vi "observacao_0MQ.vi"() -> ()   [LabVIEW 2012, in "Shared_160.lvlib"] (continued)
                n700 = call "Monta Comando.vi"("Comando"="PARAR", "Dispositivo"="PROG" ("Comando"), "Controlador"=w605) -> ()  [unwired: 4 in, 3 out]
              }
              frame 4 {
                w608 = u16 7 items=["Alarme", "Atencao", "Erro", "Ocupado", "TBD", "LCB", "Trapeira", "Paravento", "DomoRap", "DomoCW", "DomoCCW", "TBD", "Em movimento", "TBD"] ("NomeStatus")
                # "Verifica Paravento"
                n701 = call "Bit Status CUP.vi"("NomeStatus"=w608) -> ("StatBit"=w612:bool)
                n702 = Not(x=w612) -> (.not. x?=w613:bool)
                n703 = And(x=w613, y="ChkWindDown") -> (x .and. y?=w610:bool)
                n704 = case shown="True" w610 {
                  tunnel: w609 -> [_ w616]
                  tunnel: [6 w615] -> w607
                  frame False {
                    # "Paravento abaixado\nou desabilitado"
                  }
                  frame True {
                    # "Descer Parav."
                    n705 = case shown="True" w616 {
                      tunnel: [5 w621] -> w615
                      frame False {
                        w620 = u16 4 items=["ZERO", "AH", "DEC", "TUBO", "CUP"] ("Controlador")
                        # "Aguardar abaixa/o Parav."
                        # "CLP Pronto"
                        n706 = call "Monta Comando.vi"("Comando"="DESCER", "Dispositivo"="PARAVENTO" ("Comando"), "Controlador"=w620) -> ()  [unwired: 4 in, 3 out]
                      }
                      frame True {
                        # "CLP Busy"
                        n707 = local read "TimeoutCUP"() -> (w623:u32)
                        n708 = call "TickTimeout.vi"("msInicial"=w623, "msTimeout"=u32 5000) -> ("Timeout"=w622:bool)  [unwired: 2 out]
                        n709 = case shown="True" w622 {
                          tunnel: [4 3] -> w621
                          frame False {
                          }
                          frame True {
                          }
                        }
                      }
                    }
                  }
                }
              }
              frame 5 {
                w627 = u16 7 items=["Alarme", "Atencao", "Erro", "Ocupado", "TBD", "LCB", "Trapeira", "Paravento", "DomoRap", "DomoCW", "DomoCCW", "TBD", "Em movimento", "TBD"] ("NomeStatus")
                # "Aqui também caberia um Timeout?"
                # "Também poderia ser testado o bit \"Em movimento\".\nNeste caso o código do \"IF\" deve ser permutado."
                # "Aguarda abaixamento Paravento"
                n710 = call "Bit Status CUP.vi"("NomeStatus"=w627) -> ("StatBit"=w629:bool)
                n711 = case shown="True" w629 {
                  tunnel: [5 6] -> w628
                  frame False {
                    # "Ainda movendo...\nAGUARDAR"
                  }
                  frame True {
                    # "Paravento abaixado."
                  }
                }
              }
              frame 6 {
                w632 = u16 6 items=["Alarme", "Atencao", "Erro", "Ocupado", "TBD", "LCB", "Trapeira", "Paravento", "DomoRap", "DomoCW", "DomoCCW", "TBD", "Em movimento", "TBD"] ("NomeStatus")
                # "Verifica Trapeira"
                n712 = call "Bit Status CUP.vi"("NomeStatus"=w632) -> ("StatBit"=w633:bool)
                n713 = Not(x=w633) -> (.not. x?=w637:bool)
                n714 = And(x=w637, y="ChkOpenShutter") -> (x .and. y?=w635:bool)
                n715 = case shown="False" w635 {
                  tunnel: [0 w642] -> w638
                  tunnel: w634 -> [_ w643]
                  frame False {
                    # "Verificar Paravento"
                    # "Trapeira aberta\nou desabilitada"
                    n716 = call "TickTimeout.vi"() -> ("msTick"=w639:u32)  [unwired: 2 in, 2 out]
                    n717 = local write "TimeoutCUP"(w639) -> ()
                    n718 = global write "Global_Telescopio.vi" "T cup"(w639) -> ()
                    "Dome on Target" <- TRUE
                  }
                  frame True {
                    # "Abrir Trapeira"
                    n719 = case shown="False" w643 {
                      tunnel: [7 w648] -> w642
                      frame False {
                        w647 = u16 4 items=["ZERO", "AH", "DEC", "TUBO", "CUP"] ("Controlador")
                        # "Aguardar abertura Trap."
                        # "CLP Pronto"
                        n720 = call "Monta Comando.vi"("Comando"="ABRIR", "Dispositivo"="TRAPEIRA" ("Comando"), "Controlador"=w647) -> ()  [unwired: 4 in, 3 out]
                      }
                      frame True {
                        # "CLP Busy"
                        n721 = local read "TimeoutCUP"() -> (w650:u32)
                        n722 = call "TickTimeout.vi"("msInicial"=w650, "msTimeout"=u32 5000) -> ("Timeout"=w649:bool)  [unwired: 2 out]
                        n723 = case shown="True" w649 {
                          tunnel: [6 3] -> w648
                          frame False {
                          }
                          frame True {
                          }
                        }
                      }
                    }
                  }
                }
              }
              frame 7 {
                w654 = u16 6 items=["Alarme", "Atencao", "Erro", "Ocupado", "TBD", "LCB", "Trapeira", "Paravento", "DomoRap", "DomoCW", "DomoCCW", "TBD", "Em movimento", "TBD"] ("NomeStatus")
                # "Aqui também caberia um Timeout?"
                # "Aguarda abertura Trapeira"
                # "Também poderia ser testado o bit \"Em movimento\".\nNeste caso o código do \"IF\" deve ser permutado."
                n724 = call "Bit Status CUP.vi"("NomeStatus"=w654) -> ("StatBit"=w655:bool)
                n725 = case shown="True" w655 {
                  tunnel: [7 0] -> w656
                  frame False {
                    # "Ainda movendo...\nAGUARDAR"
                  }
                  frame True {
                    w659 = TRUE ("Dome on Target")
                    # "Trapeira aberta.\nFIM"
                    n726 = call "TickTimeout.vi"() -> ("msTick"=w658:u32)  [unwired: 2 in, 2 out]
                    n727 = local write "Dome on Target"(w659) -> ()
                    n728 = local write "RefreshShutterState"(w659) -> ()
                    n729 = local write "TimeoutCUP"(w658) -> ()
                    n730 = global write "Global_Telescopio.vi" "T cup"(w658) -> ()
                  }
                }
              }
            }
            n731 = And(x=w523, y=w508) -> (x .and. y?=w519:bool)
            n732 = case shown="True" w519 {
              tunnel: w508 -> [w537 _]
              tunnel: [w536 "POINT" ("Boolean Text.Text")] -> w507
              frame False {
                n733 = case shown="True" w537 {
                  tunnel: ["POINT" ("Boolean Text.Text") "STOP" ("Boolean Text.Text")] -> w536
                  frame False {
                  }
                  frame True {
                  }
                }
              }
              frame True {
                w540 = TRUE
                # "MUDANÇA:\n22/6/2011 \nHab. Guider"
                n734 = local read "ChkDomeEnable"() -> (w541:bool)
                n735 = global write "Global_Telescopio.vi" "Botão GO = STOP"(FALSE) -> ()
                n736 = local write "LED GUIDER"(w540) -> ()
                n737 = local write "GUIDER"(w540) -> ()
                n738 = local write "DOME"(w541) -> ()
              }
            }
            n739 = Tick Count (ms)() -> (millisecond timer value=w500:u32)
            n740 = Subtract(x=w500, y=w506) -> (x-y=w499:u32)
            n741 = Less?(x=w499, y=w501) -> (x < y?=w502:bool)
            n742 = case shown="True" w502 {
              tunnel: w501 -> [_ w535]
              frame False {
              }
              frame True {
                n743 = Wait Until Next ms Multiple(millisecond multiple=w535) -> ()  [unwired: 1 out]
              }
            }
            n744 = control-ref of="BtTargetPoint"() -> (w534:refnum<vi>)
            n745 = call "PROTECAO.vi"("Estado In"=w512) -> ("Estado Out"=w511:i32)  [unwired: 2 in]
            n746 = property class="Bool"(reference=w534, "Boolean Text.Text"=w507) -> ()  [unwired: 1 in, 2 out]
            n747 = local write "statCUP"(w511) -> ()
            "statCUP 2" <- "statCUP"
            "Erro Lim" <- 15 ("y")
            "Erro PROTEC" <- 10 ("y")
          }
          frame #4 {
            # "CHECA FINAL DO APONTAMENTO"
            # "ascensão reta = tempo sideral - ângulo horário (2)"
            n748 = local read "LedPointing"() -> (w957:bool)
            n749 = case shown="True" w957 {
              frame False {
                n750 = property on="DOME" class="Bool (strict)"("Disabled"=u8 0) -> ()  [unwired: 2 in, 2 out]
              }
              frame True {
                n751 = local read "statCUP"() -> (w962:i32)
                n752 = local read "statAH"() -> (w961:i32)
                n753 = local read "statDEC"() -> (w963:i32)
                n754 = Compound Arithmetic op=ADD(w962, w961, w963) -> (w964:i32)
                n755 = Greater Than 0?(x=w964) -> (x > 0?=w960:bool)
                n756 = case shown="False" w960 {
                  selector: w960 -> [w965 _]
                  frame False {
                    w968 = TRUE
                    n757 = local read "ChkPointPrecessed"() -> (w966:bool)
                    n758 = local read "StrPointObjName"() -> (w971:string)
                    n759 = local read "StrPointObjRA"() -> (w970:string)
                    n760 = local read "StrPointObjDEC"() -> (w969:string)
                    n761 = local write "LedPointing"(w965) -> ()
                    n762 = property on="LedPointing" class="Bool (strict)"("Visible"=w965) -> ()  [unwired: 2 in, 2 out]
                    n763 = case shown="True" w966 {
                      tunnel: ["2000.000000000" ("Saída") w973] -> w967
                      frame False {
                        # "20240805"
                      }
                      frame True {
                        # "20240805"
                        n764 = call "Calcula epoch.vi"() -> ("epoch"=w976:dbl)  [unwired: 2 in]
                        n765 = Number To Fractional String(number=w976, precision (6)=i16 9) -> (F-format string=w974:string)  [unwired: 2 in]
                        n766 = call "Comma_to_Point.vi"("Lat_A"=w974) -> ("Saída"=w973:string)
                      }
                    }
                    n767 = global write "Global_Telescopio.vi" "NAME OBJETO"(w971) -> ()
                    n768 = global write "Global_Telescopio.vi" "DEC AQUIS"(w969) -> ()
                    n769 = global write "Global_Telescopio.vi" "RA AQUIS"(w970) -> ()
                    n770 = local write "Processa Centragem"(w968) -> ()
                    n771 = property on="LedPointWorkArea" class="Bool (strict)"("Visible"=w968) -> ()  [unwired: 2 in, 2 out]
                    n772 = global write "Global_Telescopio.vi" "EPOCH AQUIS"(w967) -> ()
                  }
                  frame True {
                  }
                }
              }
            }
            n773 = local read "VARIABLE \nTRACKING"() -> (w958:bool)
            n774 = case shown="True" w958 {
              frame False {
              }
              frame True {
                n775 = local write "DEC"("DECTARGET") -> ()
                n776 = local write "RA"("AHTARGET") -> ()
              }
            }
          }
          frame #5 {
            # "PROCESSO OBJETO CENTRADO"
            n777 = case shown="True" "Processa Centragem" {
              frame False {
              }
              frame True {
                w985 = u16 3 items=["Alarme", "Atencao", "Erro", "Ocupado", "Protecao", "Embreagem", "Tracking", "Var. Track", "Rápido", "Ligeiro", "Médio", "Lento", "Em movimento", ""] ("NomeStatus")
                w986 = u16 3 items=["Alarme", "Atencao", "Erro", "Ocupado", "Protecao", "Embreagem", "Tracking", "Var. Track", "Rápido", "Ligeiro", "Médio", "Lento", "Em movimento", ""] ("NomeStatus")
                # "Roda case interno quando \nos controladores AH e DEC\nestiverem desocupados."
                n778 = call "Bit Status AH.vi"("NomeStatus"=w986) -> ("StatBit"=w984:bool)
                n779 = call "Bit Status DEC.vi"("NomeStatus"=w985) -> ("StatBit"=w983:bool)
                n780 = Or(x=w984, y=w983) -> (x .or. y?=w980:bool)
                n781 = case shown="False" w980 {
                  selector: w980 -> [w1005 _]
                  tunnel: "INDEXER" ("Comando") -> [w1007 _]
                  tunnel: "ZERAR" ("Comando") -> [w1006 _]
                  frame False {
                    w993 = u16 1 items=["ZERO", "AH", "DEC", "TUBO", "CUP"] ("Controlador")
                    w994 = u16 2 items=["ZERO", "AH", "DEC", "TUBO", "CUP"] ("Controlador")
                    w987 = 0.0 ("AcumAG DEC")
                    # "PROCESSOPRECESSÃO"
                    # "PROCESSO ZERA POS_MOTOR"
                    # "Precessão"
                    n782 = local read "PM_RA"() -> (w999:string)
                    n783 = local read "Temp amb"() -> (w1002:string)
                    n784 = local read "hum local"() -> (w1000:string)
                    n785 = local read "MeanDEC"() -> (w1003:string)
                    n786 = local read "pressão atm"() -> (w1001:string)
                    n787 = local read "MeanRA"() -> (w1004:string)
                    n788 = local read "PM_DEC"() -> (w998:string)
                    n789 = call "Monta Comando.vi"("Comando"=w1006, "Dispositivo"=w1007, "Controlador"=w993) -> ()  [unwired: 4 in, 3 out]
                    n790 = call "Monta Comando.vi"("Comando"=w1006, "Dispositivo"=w1007, "Controlador"=w994) -> ()  [unwired: 4 in, 3 out]
                    n791 = call "PrecessFortran.vi"("Asc reta"=w1004, "Var RA"=w999, "Declinação"=w1003, "Temperatura (Kelvin)"=w1002, "Pressao atmosferica (mB)"=w1001, "Humidade relativa (0 a 1)"=w1000, "Var DEC"=w998) -> ("Observed RA (radians)"=w997:dbl, "Observed Dec (radians)"=w996:dbl)  [unwired: 2 in, 5 out]
                    n792 = local write "Processa Centragem"(w1005) -> ()
                    n793 = global write "Global_Telescopio.vi" "LatchPrecRA"(w997) -> ()
                    n794 = global write "Global_Telescopio.vi" "LatchPrecDEC"(w996) -> ()
                    n795 = global read "Global_Telescopio.vi" "Sideral Time"() -> (w990:dbl)
                    n796 = global read "Global_Telescopio.vi" "PosDEC"() -> (w992:dbl)
                    n797 = global read "Global_Telescopio.vi" "PosAH"() -> (w991:dbl)
                    n798 = Subtract(x=w990, y=w991) -> (x-y=w989:dbl)
                    n799 = local write "LatchDeslocDEC"(w992) -> ()
                    n800 = local write "LatchDeslocRA"(w989) -> ()
                    n801 = global write "Global_Telescopio.vi" "AcumPrecDEC"(w987) -> ()
                    n802 = global write "Global_Telescopio.vi" "LatchAG RA"(w987) -> ()
                    n803 = global write "Global_Telescopio.vi" "AcumAG DEC"(w987) -> ()
                    n804 = global write "Global_Telescopio.vi" "AcumPrecRA"(w987) -> ()
                    n805 = global write "Global_Telescopio.vi" "LatchAG DEC"(w987) -> ()
                    n806 = global write "Global_Telescopio.vi" "AcumAG RA"(w987) -> ()
                    n807 = global write "Global_Telescopio.vi" "ObjCentrado"(TRUE) -> ()
                    n808 = property on="Calagem" class="Bool"("Disabled"=u8 0) -> ()  [unwired: 2 in, 2 out]
                  }
                  frame True {
                  }
                }
              }
            }
          }
          frame #6 {
            w1011 = u16 2 items=["Alarme", "Atencao", "Erro", "Ocupado", "TBD", "LCB", "Trapeira", "Paravento", "DomoRap", "DomoCW", "DomoCCW", "TBD", "Em movimento", "TBD"] ("NomeStatus")
            w1012 = u16 3 items=["Alarme", "Atencao", "Erro", "Ocupado", "TBD", "LCB", "Trapeira", "Paravento", "DomoRap", "DomoCW", "DomoCCW", "TBD", "Em movimento", "TBD"] ("NomeStatus")
            w1016 = u16 3 items=["Alarme", "Atencao", "Erro", "Ocupado", "Protecao", "Embreagem", "Tracking", "Var. Track", "Rápido", "Ligeiro", "Médio", "Lento", "Em movimento", ""] ("NomeStatus")
            w1017 = u16 3 items=["Alarme", "Atencao", "Erro", "Ocupado", "Protecao", "Embreagem", "Tracking", "Var. Track", "Rápido", "Ligeiro", "Médio", "Lento", "Em movimento", ""] ("NomeStatus")
            w1025 = "ERROS" ("Comando")
            w1028 = u16 2 items=["Alarme", "Atencao", "Erro", "Ocupado", "Protecao", "Embreagem", "Tracking", "Var. Track", "Rápido", "Ligeiro", "Médio", "Lento", "Em movimento", ""] ("NomeStatus")
            w1029 = u16 2 items=["Alarme", "Atencao", "Erro", "Ocupado", "Protecao", "Embreagem", "Tracking", "Var. Track", "Rápido", "Ligeiro", "Médio", "Lento", "Em movimento", ""] ("NomeStatus")
            w1026 = "PROG" ("Comando")
            # "LOGTCS ERROS"
            n809 = call "Bit Status AH.vi"("NomeStatus"=w1029) -> ("StatBit"=w1019:bool)
            n810 = call "Bit Status AH.vi"("NomeStatus"=w1017) -> ("StatBit"=w1015:bool)
            n811 = call "Bit Status DEC.vi"("NomeStatus"=w1028) -> ("StatBit"=w1018:bool)
            n812 = call "Bit Status DEC.vi"("NomeStatus"=w1016) -> ("StatBit"=w1014:bool)
            n813 = call "Bit Status CUP.vi"("NomeStatus"=w1011) -> ("StatBit"=w1027:bool)
            n814 = call "Bit Status CUP.vi"("NomeStatus"=w1012) -> ("StatBit"=w1024:bool)
            n815 = Not(x=w1024) -> (.not. x?=w1023:bool)
            n816 = Not(x=w1015) -> (.not. x?=w1021:bool)
            n817 = Not(x=w1014) -> (.not. x?=w1022:bool)
            n818 = And(x=w1027, y=w1023) -> (x .and. y?=w1010:bool)
            n819 = And(x=w1019, y=w1021) -> (x .and. y?=w1020:bool)
            n820 = And(x=w1018, y=w1022) -> (x .and. y?=w1013:bool)
            n821 = And(x=FALSE, y=w1010) -> (x .and. y?=w1009:bool)
            n822 = case shown="True" w1013 {
              selector: w1013 -> [_ w1038]
              tunnel: w1026 -> [_ w1039]
              tunnel: w1025 -> [_ w1035]
              frame False {
              }
              frame True {
                w1036 = u16 2 items=["ZERO", "AH", "DEC", "TUBO", "CUP"] ("Controlador")
                n823 = call "Monta Comando.vi"("Comando"=w1035, "Dispositivo"=w1039, "Controlador"=w1036) -> ("Resposta"=w1037:string)  [unwired: 4 in, 2 out]
                n824 = call "Envia LOG.vi"("Error message"=w1037, "Controlador"=w1036, "Log de erro"=w1038) -> ()  [unwired: 5 in, 2 out]
              }
            }
            n825 = case shown="True" w1009 {
              selector: w1009 -> [_ w1033]
              tunnel: w1026 -> [_ w1034]
              tunnel: w1025 -> [_ w1030]
              frame False {
              }
              frame True {
                w1031 = u16 4 items=["ZERO", "AH", "DEC", "TUBO", "CUP"] ("Controlador")
                n826 = call "Monta Comando.vi"("Comando"=w1030, "Dispositivo"=w1034, "Controlador"=w1031) -> ("Resposta"=w1032:string)  [unwired: 4 in, 2 out]
                n827 = call "Envia LOG.vi"("Error message"=w1032, "Controlador"=w1031, "Log de erro"=w1033) -> ()  [unwired: 5 in, 2 out]
              }
            }
            n828 = case shown="True" w1020 {
              selector: w1020 -> [_ w1043]
              tunnel: w1026 -> [_ w1044]
              tunnel: w1025 -> [_ w1040]
              frame False {
              }
              frame True {
                w1041 = u16 1 items=["ZERO", "AH", "DEC", "TUBO", "CUP"] ("Controlador")
                n829 = call "Monta Comando.vi"("Comando"=w1040, "Dispositivo"=w1044, "Controlador"=w1041) -> ("Resposta"=w1042:string)  [unwired: 4 in, 2 out]
                n830 = call "Envia LOG.vi"("Error message"=w1042, "Controlador"=w1041, "Log de erro"=w1043) -> ()  [unwired: 5 in, 2 out]
              }
            }
          }
          frame #7 {
            # "MASSA DE AR"
            # "z'"
            # "z * (1 - 0,0012* (z* z -1) )"
            # "(z* z -1)"
            # "z"
            # "O Hour Angle é calculado com essa equação (AH = TS - RA), \nsendo TS o tempo sideral que você fica calculando o tempo todo e RA a \ncoordenada que vem do quadro TARGET da aba POINTING."
            # "Coslat"
            # "Sinlat"
            # "MASSA DE AR\n# define LAT -22,534444444444 / / Lat itude do telescópio\n# define SINLAT -0,383238771 / / Seno da Lat itude\n# define COSLAT 0,923649308 / / Cosseno da Lat itude\ndouble airmass (double ah, double delta) / / ângulos dos eixos AH e DEC em radianos\n{ double z;\nz = 1./ (SINLAT* sin(delta) + COSLAT* cos(delta) * cos(ah) ) ;\nz = z * (1 - 0,0012* (z* z -1) ) ;\nif (z > = 10) z = 9.999;\nif (z < 0) z = 0;\nreturn (z) ;\n}"
            n831 = global read "Global_Telescopio.vi" "AH_now"() -> (w1045:dbl)
            n832 = global read "Global_Telescopio.vi" "delta_now"() -> (w1046:dbl)
            n833 = Cosine(x=w1046) -> (cos(x)=w1066:dbl)
            n834 = Sine(x=w1046) -> (sin(x)=w1068:dbl)
            n835 = Cosine(x=w1045) -> (cos(x)=w1064:dbl)
            n836 = Multiply(x=0.923649308 ("Delta=DEC"), y=w1066) -> (x*y=w1065:dbl)
            n837 = Multiply(x=-0.383238771 ("Delta=DEC"), y=w1068) -> (x*y=w1063:dbl)
            n838 = Multiply(x=w1065, y=w1064) -> (x*y=w1062:dbl)
            n839 = Add(x=w1063, y=w1062) -> (x+y=w1061:dbl)
            n840 = Reciprocal(x=w1061) -> (1/x=w1053:dbl)
            n841 = Subtract(x=w1053, y=1.0) -> (x-y=w1059:dbl)
            n842 = Multiply(x=w1053, y=w1059) -> (x*y=w1058:dbl)
            n843 = Multiply(x=w1058, y=0.0012) -> (x*y=w1055:dbl)
            n844 = Subtract(x=1.0 ("y"), y=w1055) -> (x-y=w1054:dbl)
            n845 = Multiply(x=w1053, y=w1054) -> (x*y=w1050:dbl)
            n846 = Greater Or Equal?(x=w1050, y=10.0) -> (x >= y?=w1051:bool)
            n847 = case shown="True" w1051 {
              tunnel: [w1072 9.999999 ("y")] -> w1048
              tunnel: w1050 -> [w1072 _]
              frame False {
              }
              frame True {
              }
            }
            n848 = Less Than 0?(x=w1048) -> (x < 0?=w1049:bool)
            n849 = case shown="True" w1049 {
              tunnel: [w1070 0.0 ("y")] -> w1047
              tunnel: w1048 -> [w1070 _]
              frame False {
              }
              frame True {
              }
            }
            "Air Mass" <- w1047
            n850 = global write "Global_Telescopio.vi" "Air Mass"(w1047) -> ()
          }
          frame #8 {
          }
          frame #9 {
            # "ZeroMQ"
            # "Atribuição \nsem efeito"
            # "CONDIÇÕES ATMOSFÉRICAS"
            # "A cada n Segundos\nEssa rotina gera 1\npulso!"
            # "Seg"
            # "Janela Das Condições Atmosféricas"
            n851 = global read "Global_Telescopio.vi" "Default Met"() -> (w1078:bool)
            n852 = local write "Default Met"(w1078) -> ()
            n853 = call "timepulse.vi"("de quantos segundos"=i16 10) -> ("PULSO"=w1077:bool)  [unwired: 2 in]
            n854 = call "Pulso_se_Mudou.vi"("Entrada"="Int/Ext") -> ("Saída"=w1075:bool)
            n855 = And(x="Int/Ext", y=w1077) -> (x .and. y?=w1074:bool)
            n856 = case shown="True" w1074 {
              tunnel: [_ TRUE ("Int/Ext")] -> w1079
              tunnel: w1075 -> [w1082 _]
              frame False {
                # "A chave Int/Ext mudou\npara pushbutton e é tratada apenas dentro deste case \"False\" nos períodos inativos de \"time pulse\" ligado ao terminal ? do case.\n\nOs valores internos (dew point, temperatura, umidade ) somente são mostrados enquanto a chave ficar pressionada pelo mouse.\n\nIsto garante o uso dos valores externos desssas grandezas no cálculo da precessão."
                n857 = case shown="False" w1082 {
                  frame False {
                  }
                  frame True {
                    # "ZeroMQ"
                    # "Display"
                    # "ESTE CASO SOMENTE É EXECUTADO QUANDO A CHAVE INT/EXT MUDA DE ESTADO"
                    n858 = local read "Int/Ext"() -> (w1087:bool)
                    n859 = case shown="True" w1087 {
                      tunnel: [28 ("index") 5 ("index")] -> w1085
                      tunnel: [29 ("index") 6 ("index")] -> w1086
                      tunnel: [27 ("index") 2 ("index")] -> w1084
                      frame False {
                        # "Interno"
                      }
                      frame True {
                        # "Externo"
                      }
                    }
                    n860 = call "Leitura Weather160.vi"() -> ("Array"=w1083:string[])  [unwired: 4 in, 1 out]
                    n861 = Index Array(array=w1083, index #1=w1084, index #2=w1085, index #3=w1086) -> (element #1=w1090:string, element #2=w1089:string, element #3=w1088:string)
                    n862 = call "point_to_comma.vi"("Lat_A"=w1090) -> ("Saída"=w1092:string)
                    n863 = call "point_to_comma.vi"("Lat_A"=w1089) -> ("Saída"=w1093:string)
                    n864 = call "point_to_comma.vi"("Lat_A"=w1088) -> ("Saída"=w1096:string)
                    n865 = Fract/Exp String To Number(string=w1092, default (0 dbl)=1.0 ("default (0 DBL)")) -> (number=w1097:dbl)  [unwired: 2 in, 1 out]
                    n866 = Fract/Exp String To Number(string=w1093, default (0 dbl)=1.0 ("default (0 DBL)")) -> (number=w1098:dbl)  [unwired: 2 in, 1 out]
                    n867 = Fract/Exp String To Number(string=w1096, default (0 dbl)=1.0 ("default (0 DBL)")) -> (number=w1099:dbl)  [unwired: 2 in, 1 out]
                    n868 = local write "Temperature"(w1097) -> ()
                    n869 = local write "Humidity"(w1098) -> ()
                    n870 = local write "Dew Point"(w1099) -> ()
                  }
                }
              }
              frame True {
                n871 = stacked-sequence {
                  frame #0 {
                    # "O botão INT/ EXT (cf. figura 3) seleciona se os most radores TEMPERATURE, HUMIDITY\ne DEW POINT são atualizados com os valores internos ou externos desse regist ro.\nA barra gráfica CLOUSURE LIMITS deve ser deslocada em função da proximidade\n(dada por um valor percentural de zero a 100%) dos valores lidos do arquivo de dados\natmosféricos com os valores- limite das grandezas listadas nesse quadro. Para\nPRESSURE e WIND SPEED, considerar os valores- limite desse quadro como o final de\numa escala de 0 a 100%, cujo valor inicial (0%) corresponde ao valor zero dessas\ngrandezas. Para as grandezas DEWPOINT, interna e externa, considerar os valores\nlimites listados no quadro como final da escala (100%) e cada décimo de ºC acima\ndos valores- limite como 1% da escala."
                    # "A simulação da janela ENVIRONMENT STATUS será feita com os dados de um arquivo\ngerado pela estação meteorológica contendo os regist ros de 24 horas de monitoria,\nsendo cada regist ro efetuado em intervalos de 10 minutos. A simulação deve procurar\nnesse arquivo (anexo, LNA-TCSPD-MP-00012-01-100.txt ) o regist ro correspondente à\nhora local do PC, ler esse regist ro e ret irar as informações de cada most rador para\natualizar essa janela."
                  }
                  frame #1 {
                    (unwired) "1:04" ("Hora a ser Procurada")
                    w1130 = "\t"
                    # "ZeroMQ"
                    # "ZeroMQ"
                    # "Formato"
                    # "MUDANÇA FUTURA:\nSe possível, mostrar os valores de Pressão atm,\nTemp. amb. e umidade rel.\nda estação do tubo em lugar\ndos valores internos."
                    # "O Fortran usa valores\nde umidade entre 0 e 1."
                    # "MUDANÇA 08/04/2011:\nCriada a variável AtmosferaStr para guardar dados\nmeteorológicos para Erros de Apontamento"
                    # "Celsius -->Kelvin\nO Fortran usa Kelvin"
                    # "bar"
                    n872 = case shown="True" TRUE {
                      tunnel: [27 ("index") 2 ("index")] -> w1123
                      tunnel: [28 ("index") 5 ("index")] -> w1122
                      tunnel: [29 ("index") 6 ("index")] -> w1121
                      frame False {
                        # "Interno"
                      }
                      frame True {
                        # "Externo"
                      }
                    }
                    n873 = case shown="True" "Default Met" {
                      tunnel: ["OFF" "ON"] -> w1112
                      frame False {
                      }
                      frame True {
                      }
                    }
                    n874 = property on="Default" class="Str"("Visible"="Default Met") -> ()  [unwired: 2 in, 2 out]
                    n875 = global write "Global_Telescopio.vi" "WS_DEFAULT"(w1112) -> ()
                    n876 = call "Leitura Weather160.vi"() -> ("Erro de Leitura=True"=w1107:bool, "Array"=w1108:string[])  [unwired: 4 in]
                    n877 = case shown="False" "Default Met" {
                      tunnel: w1107 -> [w1175 _]
                      frame False {
                        # "."
                        n878 = local write "Default Met"(w1175) -> ()
                      }
                      frame True {
                      }
                    }
                    n879 = Index Array(array=w1108, index #1=w1123, index #2=w1122, index #3=w1121, index #4=7 ("index"), index #5=8 ("index"), index #6=12 ("index"), index #7=16 ("index"), index #8=2 ("index"), index #9=5 ("index"), index #10=27 ("index"), index #11=28 ("index"), index #12=35 ("index")) -> (element #1=w1159:string, element #2=w1172:string, element #3=w1169:string, element #4=w1165:string, element #5=w1131:string, element #6=w1164:string, element #7=w1160:string, element #8=w1143:string, element #9=w1142:string, element #10=w1141:string, element #11=w1140:string, element #12=w1125:string)
                    "Wind Dir" <- w1131
                    n880 = Decimal String To Number(string=w1125) -> (number=→"LEAF":i32)  [unwired: 2 in, 1 out]
                    n881 = call "point_to_comma.vi"("Lat_A"=w1159) -> ("Saída"=w1156:string)
                    n882 = call "point_to_comma.vi"("Lat_A"=w1172) -> ("Saída"=w1157:string)
                    n883 = call "point_to_comma.vi"("Lat_A"=w1169) -> ("Saída"=w1134:string)
                    n884 = call "point_to_comma.vi"("Lat_A"=w1165) -> ("Saída"=w1132:string)
                    n885 = call "point_to_comma.vi"("Lat_A"=w1164) -> ("Saída"=w1133:string)
                    n886 = call "point_to_comma.vi"("Lat_A"=w1160) -> ("Saída"=w1137:string)
                    "pressão atm" <- w1137
                    n887 = call "point_to_comma.vi"("Lat_A"=w1143) -> ("Saída"=w1139:string)
                    n888 = call "point_to_comma.vi"("Lat_A"=w1142) -> ("Saída"=w1138:string)
                    n889 = call "point_to_comma.vi"("Lat_A"=w1141) -> ("Saída"=w1136:string)
                    n890 = call "point_to_comma.vi"("Lat_A"=w1140) -> ("Saída"=w1135:string)
                    n891 = Concatenate Strings(w1139, w1130, w1138, w1130, w1137, w1130, w1136, w1130, w1135, w1130, w1134, w1130, w1132, w1130, w1131, w1130) -> (→"AtmosferaStr":string)
                    n892 = Fract/Exp String To Number(string=w1156, default (0 dbl)=1.0 ("default (0 DBL)")) -> (number=w1128:dbl)  [unwired: 2 in, 1 out]
                    "Temperature" <- w1128
                    n893 = Fract/Exp String To Number(string=w1157, default (0 dbl)=1.0 ("default (0 DBL)")) -> (number=w1127:dbl)  [unwired: 2 in, 1 out]
                    "Humidity" <- w1127
                    n894 = Fract/Exp String To Number(string=w1134, default (0 dbl)=1.0 ("default (0 DBL)")) -> (number=→"Dew Point":dbl)  [unwired: 2 in, 1 out]
                    n895 = Fract/Exp String To Number(string=w1132, default (0 dbl)=1.0 ("default (0 DBL)")) -> (number=→"Wind Speed":dbl)  [unwired: 2 in, 1 out]
                    n896 = Fract/Exp String To Number(string=w1133, default (0 dbl)=1.0 ("default (0 DBL)")) -> (number=→"Wind Chill":dbl)  [unwired: 2 in, 1 out]
                    n897 = Fract/Exp String To Number(string=w1137, default (0 dbl)=1.0 ("default (0 DBL)")) -> (number=w1126:dbl)  [unwired: 2 in, 1 out]
                    "Pressure" <- w1126
                    n898 = Fract/Exp String To Number(string=w1139, default (0 dbl)=1.0 ("default (0 DBL)")) -> (number=w1146:dbl)  [unwired: 2 in, 1 out]
                    n899 = Fract/Exp String To Number(string=w1138, default (0 dbl)=1.0 ("default (0 DBL)")) -> (number=w1145:dbl)  [unwired: 2 in, 1 out]
                    n900 = Add(x=w1146, y=273.5 ("default (0 DBL)")) -> (x+y=w1154:dbl)
                    n901 = Divide(x=w1145, y=100.0 ("default (0 DBL)")) -> (x/y=w1148:dbl)
                    n902 = global write "Global_Telescopio.vi" "HUM"(w1127) -> ()
                    n903 = global write "Global_Telescopio.vi" "TEMP"(w1128) -> ()
                    n904 = global write "Global_Telescopio.vi" "BAR"(w1126) -> ()
                    n905 = Number To Fractional String(number=w1154, precision (6)=i16 1) -> (F-format string=→"Temp amb":string)  [unwired: 2 in]
                    n906 = Number To Fractional String(number=w1148, precision (6)=i16 2) -> (F-format string=→"hum local":string)  [unwired: 2 in]
                  }
                  frame #2 {
                    # "Em relação as suas perguntas:\n- Temperaturas (Temperature, Dew Point e Wind Chill): mínimo/máximo: -20 a +50 graus\n- Humidity:  0 a 100%\n- Pressão atmosférica: de 300 a 1200 mBar\n- Velocidade do vento: 0 a 300 Km/h\n\nNotar que a chave INT/EXT na parte superior do quadro \nesquerdo seleciona se são mostrados os valores internos ou externos de Temperatura, Umidade e Dew Point."
                    # "Pressure Max"
                    # "Wind chill Point Max"
                    # "Temp Point Max"
                    # "Dew Point Max"
                    # "Humidity Max"
                    # "Speed Max"
                    # "Steady Wind           >  70 Km/h\nRelative Humidity    >  97 %\nInternal Dewpoint  <  0.5  C\nExternal Dewpoint <  1.0  C"
                    n907 = Divide(x=100.0, y=300.0 ("x")) -> (x/y=w1213:dbl)
                    n908 = Divide(x=100.0, y=100.0 ("x")) -> (x/y=w1207:dbl)
                    n909 = Divide(x=100.0, y=50.0 ("x")) -> (x/y=w1205:dbl)
                    n910 = Divide(x=100.0, y=50.0 ("x")) -> (x/y=w1199:dbl)
                    n911 = Divide(x=100.0, y=50.0 ("x")) -> (x/y=w1198:dbl)
                    n912 = Divide(x=100.0, y=1200.0 ("x")) -> (x/y=w1193:dbl)
                    n913 = local read "Temperature"() -> (w1190:dbl)
                    n914 = local read "Wind Speed"() -> (w1212:dbl)
                    n915 = local read "Wind Chill"() -> (w1191:dbl)
                    n916 = local read "Dew Point"() -> (w1202:dbl)
                    n917 = local read "Humidity"() -> (w1206:dbl)
                    n918 = local read "Pressure"() -> (w1192:dbl)
                    n919 = Multiply(x=w1212, y=w1213) -> (x*y=w1189:dbl)
                    n920 = Multiply(x=w1206, y=w1207) -> (x*y=w1188:dbl)
                    n921 = Multiply(x=w1202, y=w1205) -> (x*y=w1187:dbl)
                    n922 = Multiply(x=w1190, y=w1199) -> (x*y=w1186:dbl)
                    n923 = Multiply(x=w1191, y=w1198) -> (x*y=w1185:dbl)
                    n924 = Multiply(x=w1192, y=w1193) -> (x*y=w1184:dbl)
                    n925 = Build Array(w1189, w1188, w1187, w1186, w1185, w1184) -> (w1183:dbl[])
                    n926 = Array Max & Min(array=w1183) -> (max value=w1182:dbl)  [unwired: 3 out]
                    n927 = local write "SlideEnviromental"(w1182) -> ()
                  }
                  frame #3 {
                    # "Determinadas as proximidades de cada grandeza em valores percentuais, selecionar o\nvalor da mais elevada para ser most rado na barra gráfica. A cor dessa barra gráfica\ndeve mudar em função do valor most rado. Enquanto est iver abaixo de 90%, ela deve\nser verde, ent re 90 e 95% amarela e acima de 95% vermelha. O led ao lado desse\nbarra deve ficar ligado e ter a mesma cor da barra gráfica, mas quando esta\nult rapassar 90%, ou seja quando for amarela ou vermelha, o led deve piscar."
                    n928 = local read "SlideEnviromental"() -> (w1214:dbl)
                    n929 = In Range and Coerce(upper limit=95.0 ("lower limit"), x=w1214, lower limit=90.0 ("upper limit")) -> (In Range?=w1219:bool)  [unwired: 1 out]
                    n930 = Less?(x=w1214, y=90.0) -> (x < y?=w1221:bool)
                    n931 = Greater?(x=w1214, y=95.0 ("lower limit")) -> (0:w1218:bool)
                    n932 = case shown="True" w1219 {
                      frame False {
                      }
                      frame True {
                        n933 = stacked-sequence {
                          frame #0 {
                            n934 = property on="SlideEnviromental" class="Slide (strict)"("Fill Color"=u32 16772882) -> ()  [unwired: 2 in, 2 out]
                            n935 = local write "Boolean 11"(TRUE ("Boolean 11")) -> ()
                            n936 = property on="Boolean 11" class="Bool (strict)"("Blinking"=FALSE) -> ()  [unwired: 2 in, 2 out]
                          }
                          frame #1 {
                            # "Cor do Led"
                            # "lig"
                            # "des"
                            n937 = Bundle(u32 7171459, u32 46096) -> (w1241:cluster{u32, u32})  [unwired: 1 in]
                            n938 = Bundle(u32 16772882, u32 46096) -> (w1240:cluster{u32, u32})  [unwired: 1 in]
                            n939 = Build Array(w1241, w1240) -> (w1239:cluster{u32, u32}[])
                            n940 = property on="Boolean 11" class="Bool (strict)"("Colors [4]"=w1239) -> ()  [unwired: 2 in, 2 out]
                          }
                        }
                      }
                    }
                    n941 = case shown="True" w1221 {
                      frame False {
                      }
                      frame True {
                        n942 = stacked-sequence {
                          frame #0 {
                            n943 = property on="SlideEnviromental" class="Slide (strict)"("Fill Color"=u32 6618880) -> ()  [unwired: 2 in, 2 out]
                            n944 = local write "Boolean 11"(TRUE ("Boolean 11")) -> ()
                            n945 = property on="Boolean 11" class="Bool (strict)"("Blinking"=FALSE) -> ()  [unwired: 2 in, 2 out]
                          }
                          frame #1 {
                            # "Cor do Led"
                            # "lig"
                            # "des"
                            n946 = Bundle(u32 7171459, u32 46096) -> (w1245:cluster{u32, u32})  [unwired: 1 in]
                            n947 = Bundle(u32 6618880, u32 46096) -> (w1246:cluster{u32, u32})  [unwired: 1 in]
                            n948 = Build Array(w1245, w1246) -> (w1247:cluster{u32, u32}[])
                            n949 = property on="Boolean 11" class="Bool (strict)"("Colors [4]"=w1247) -> ()  [unwired: 2 in, 2 out]
                          }
                        }
                      }
                    }
                    n950 = case shown="True" w1218 {
                      frame False {
                      }
                      frame True {
                        n951 = stacked-sequence {
                          frame #0 {
                            n952 = local write "Boolean 11"(TRUE ("Boolean 11")) -> ()
                            n953 = property on="SlideEnviromental" class="Slide (strict)"("Fill Color"=u32 16715776) -> ()  [unwired: 2 in, 2 out]
                            n954 = property on="Boolean 11" class="Bool (strict)"("Blinking"=TRUE) -> ()  [unwired: 2 in, 2 out]
                          }
                          frame #1 {
                            # "Cor do Led"
                            # "lig"
                            # "des"
                            n955 = Bundle(u32 7171459, u32 46096) -> (w1225:cluster{u32, u32})  [unwired: 1 in]
                            n956 = Bundle(u32 16715776, u32 46096) -> (w1226:cluster{u32, u32})  [unwired: 1 in]
                            n957 = Build Array(w1225, w1226) -> (w1227:cluster{u32, u32}[])
                            n958 = property on="Boolean 11" class="Bool (strict)"("Colors [4]"=w1227) -> ()  [unwired: 2 in, 2 out]
                          }
                        }
                      }
                    }
                  }
                }
              }
            }
            n959 = flat-sequence {
              tunnel: w1079 -> [_]
              frame #0 {
                n960 = local read "LEAF"() -> (w1081:i32)
                n961 = call "Testa_Leaf.vi"("LEAF"=w1081) -> ()  [unwired: 11 in]
              }
            }
          }
          frame #10 {
            w1262 = u16 3 items=["Alarme", "Atencao", "Erro", "Ocupado", "Protecao", "Embreagem", "Tracking", "Var. Track", "Rápido", "Ligeiro", "Médio", "Lento", "Em movimento", ""] ("NomeStatus")
            w1263 = u16 3 items=["Alarme", "Atencao", "Erro", "Ocupado", "Protecao", "Embreagem", "Tracking", "Var. Track", "Rápido", "Ligeiro", "Médio", "Lento", "Em movimento", ""] ("NomeStatus")
            # "PROCESSO AUTO GUIDER"
            n962 = local read "MOUNT"() -> (w1259:bool)
            n963 = local read "LedPointing"() -> (w1257:bool)
            n964 = global read "Global_Telescopio.vi" "Correção Guider"() -> (w1253:bool)
            n965 = local read "MOVING"() -> (w1256:bool)
            n966 = call "Bit Status AH.vi"("NomeStatus"=w1263) -> ("StatBit"=w1260:bool)
            n967 = call "Bit Status DEC.vi"("NomeStatus"=w1262) -> ("StatBit"=w1261:bool)
            n968 = Not(x=w1256) -> (.not. x?=w1255:bool)
            n969 = Not(x=w1257) -> (.not. x?=w1254:bool)
            n970 = Not Or(1:w1261, 2:w1260) -> (0:w1258:bool)
            n971 = Compound Arithmetic op=AND(w1253, w1254, w1255, "GUIDER", w1259, w1258) -> (w1264:bool)
            n972 = case shown="True" w1264 {
              frame False {
                # "Reseta Flag da comunicação do Guider"
                n973 = global write "Global_Telescopio.vi" "Correção Guider"(FALSE ("Correção Guider")) -> ()
              }
              frame True {
                # "MUDANÇA:\n(25/08/2010)"
                # "É necessário testar se as\nstrings são igual a espaço\nem virtude de um BUG,\nno Soft do Auto guider!"
                n974 = global read "Global_Telescopio.vi" "guide_dir_ns"() -> (w1271:string)
                n975 = global read "Global_Telescopio.vi" "guide_dir_we"() -> (w1272:string)
                n976 = case shown="\"E\"" w1272 {
                  tunnel: [0.0 ("PreciseOffsetDEC 2") 1.0 ("PreciseOffsetDEC 2") -1.0 ("PreciseOffsetDEC 2")] -> w1269
                  frame " ", Default {
                  }
                  frame "W" {
                  }
                  frame "E" {
                  }
                }
                n977 = case shown="\"N\"" w1271 {
                  tunnel: [0.0 ("PreciseOffsetDEC 2") 1.0 ("PreciseOffsetDEC 2") -1.0 ("PreciseOffsetDEC 2")] -> w1268
                  frame " ", Default {
                  }
                  frame "N" {
                  }
                  frame "S" {
                  }
                }
                n978 = Equal To 0?(x=w1268) -> (x = 0?=w1267:bool)
                n979 = Equal To 0?(x=w1269) -> (x = 0?=w1266:bool)
                n980 = And(x=w1266, y=w1267) -> (x .and. y?=w1270:bool)
                n981 = case shown="False" w1270 {
                  tunnel: w1269 -> [w1277 _]
                  tunnel: w1268 -> [w1276 _]
                  frame False {
                    # "Comandos do Auto guider contendo direção"
                    n982 = global read "Global_Telescopio.vi" "esc_placa"() -> (w1275:string)
                    n983 = Fract/Exp String To Number(use system decimal point (T)=FALSE, string=w1275) -> (number=w1274:dbl)  [unwired: 2 in, 1 out]
                    n984 = stacked-sequence {
                      tunnel: w1277 -> [w1283 _ _]
                      tunnel: w1276 -> [_ w1303 _]
                      tunnel: w1274 -> [w1280 w1300 _]
                      frame #0 {
                        n985 = local read "AtualDEC"() -> (w1288:dbl)
                        n986 = global read "Global_Telescopio.vi" "CorrecaoMin"() -> (w1278:dbl)
                        n987 = global read "Global_Telescopio.vi" "guide_asc"() -> (w1282:dbl)
                        n988 = Cosine(x=w1288) -> (cos(x)=w1287:dbl)
                        n989 = Multiply(x=w1282, y=w1280) -> (x*y=w1281:dbl)
                        n990 = Absolute Value(x=w1287) -> (abs(x)=w1286:dbl)
                        n991 = Divide(x=w1281, y=w1286) -> (x/y=w1284:dbl)
                        n992 = Multiply(x=w1283, y=w1284) -> (x*y=w1279:dbl)
                        n993 = Greater?(x=w1284, y=w1278) -> (0:w1285:bool)
                        n994 = case shown="True" w1285 {
                          tunnel: w1279 -> [_ w1290]
                          frame False {
                          }
                          frame True {
                            w1294 = u16 1 items=["ZERO", "AH", "DEC", "TUBO", "CUP"] ("Controlador")
                            # "PROCESSO MOVE TELESCÓPIO"
                            n995 = local read "Offset RA"() -> (w1291:dbl)
                            n996 = Add(x=w1290, y=w1291) -> (x+y=w1292:dbl)
                            n997 = property on="Calagem" class="Bool"("Disabled"=u8 2) -> ()  [unwired: 2 in, 2 out]
                            n998 = call "Conversao Ms to Hora texto.vi"("TRUE=HORA\nFALSE=GRAU"=TRUE ("TRUE=HORA\nFALSE=GRAU"), "PrecDEC"=w1290) -> ("Hora/Graus Texto Decimal"=w1297:string)
                            n999 = local write "Offset RA"(w1292) -> ()
                            n1000 = call "Monta Comando.vi"("Set Point"=w1297, "Comando"="MOVER_REL", "Dispositivo"="EIXO" ("Comando"), "Controlador"=w1294) -> ()  [unwired: 3 in, 3 out]
                          }
                        }
                      }
                      frame #1 {
                        n1001 = global read "Global_Telescopio.vi" "guide_dec"() -> (w1302:dbl)
                        n1002 = Multiply(x=w1302, y=w1300) -> (x*y=w1301:dbl)
                        n1003 = global read "Global_Telescopio.vi" "CorrecaoMin"() -> (w1298:dbl)
                        n1004 = Greater?(x=w1301, y=w1298) -> (0:w1304:bool)
                        n1005 = Multiply(x=w1303, y=w1301) -> (x*y=w1299:dbl)
                        n1006 = case shown="True" w1304 {
                          tunnel: w1299 -> [_ w1306]
                          frame False {
                          }
                          frame True {
                            w1310 = u16 2 items=["ZERO", "AH", "DEC", "TUBO", "CUP"] ("Controlador")
                            # "PROCESSO MOVE TELESCÓPIO"
                            n1007 = local read "Offset DEC"() -> (w1307:dbl)
                            n1008 = Add(x=w1306, y=w1307) -> (x+y=w1308:dbl)
                            n1009 = property on="Calagem" class="Bool"("Disabled"=u8 2) -> ()  [unwired: 2 in, 2 out]
                            n1010 = call "Conversao Ms to Hora texto.vi"("TRUE=HORA\nFALSE=GRAU"=FALSE ("TRUE=HORA\nFALSE=GRAU"), "PrecDEC"=w1306) -> ("Hora/Graus Texto Decimal"=w1313:string)
                            n1011 = local write "Offset DEC"(w1308) -> ()
                            n1012 = call "Monta Comando.vi"("Set Point"=w1313, "Comando"="MOVER_REL", "Dispositivo"="EIXO" ("Comando"), "Controlador"=w1310) -> ()  [unwired: 3 in, 3 out]
                          }
                        }
                      }
                      frame #2 {
                        # "Reseta Flag da comunicação do Guider"
                        n1013 = global write "Global_Telescopio.vi" "Correção Guider"(FALSE ("Correção Guider")) -> ()
                      }
                    }
                  }
                  frame True {
                  }
                }
              }
            }
            "LED GUIDER" <- "GUIDER"
          }
          frame #11 {
            w1330 = u16 12 items=["Alarme", "Atencao", "Erro", "Ocupado", "Protecao", "Embreagem", "Tracking", "Var. Track", "Rápido", "Ligeiro", "Médio", "Lento", "Em movimento", ""] ("NomeStatus")
            w1329 = u16 12 items=["Alarme", "Atencao", "Erro", "Ocupado", "Protecao", "Embreagem", "Tracking", "Var. Track", "Rápido", "Ligeiro", "Médio", "Lento", "Em movimento", ""] ("NomeStatus")
            # "Aqui era a Global\nLIMITE"
            # "Este teste deve ser executado antes do Frame de enviar\ncomando do sistema de aquisição, em virtude de teste do \nmovimento."
            # "Quando o Movimento Parar\nreseta a Variável/Flag para enviar \no CR ao sitema de Aquisição"
            n1014 = global read "Global_Telescopio.vi" "AQ Offset Mov"() -> (w1326:bool)
            n1015 = call "Bit Status AH.vi"("NomeStatus"=w1329) -> ("StatBit"=w1332:bool)
            n1016 = call "Bit Status DEC.vi"("NomeStatus"=w1330) -> ("StatBit"=w1331:bool)
            n1017 = local read "Proteção"() -> (w1322:bool)
            n1018 = Not Or(1:w1331, 2:w1332) -> (0:w1327:bool)
            n1019 = case shown="True" w1322 {
              selector: w1322 -> [w1333 w1334]
              frame False {
                n1020 = local write "LIMITE"(w1333) -> ()
                n1021 = property on="LIMITE" class="Bool"("Blinking"=w1333) -> ()  [unwired: 2 in, 2 out]
              }
              frame True {
                n1022 = property on="LIMITE" class="Bool"("Blinking"=w1334) -> ()  [unwired: 2 in, 2 out]
                "LIMITE" <- w1334
              }
            }
            n1023 = And(x=w1326, y=w1327) -> (x .and. y?=w1328:bool)
            n1024 = case shown="True" w1328 {
              frame False {
              }
              frame True {
                n1025 = global write "Global_Telescopio.vi" "AQ Offset Mov"(FALSE ("AQ Offset Mov")) -> ()
              }
            }
            n1026 = global read "Global_Telescopio.vi" "Z_SEGURANÇA_GRAUS"() -> (w1325:dbl)
            n1027 = global read "Global_Telescopio.vi" "Zenital angle GRAUS"() -> (w1324:dbl)
            n1028 = global read "Global_Telescopio.vi" "FinalsFileDownload"() -> (→"Precess Data out-of-date":bool)
            n1029 = Greater?(x=w1324, y=w1325) -> (0:→"Security Zone":bool)
          }
          frame #12 {
            w1349 = u16 8 items=["Alarme", "Atencao", "Erro", "Ocupado", "Protecao", "Embreagem", "Tracking", "Var. Track", "Rápido", "Ligeiro", "Médio", "Lento", "Em movimento", ""] ("NomeStatus")
            w1350 = u16 8 items=["Alarme", "Atencao", "Erro", "Ocupado", "Protecao", "Embreagem", "Tracking", "Var. Track", "Rápido", "Ligeiro", "Médio", "Lento", "Em movimento", ""] ("NomeStatus")
            # "ATUALIZAÇÃO DO QUADRO STATUS INFORMATION"
            n1030 = call "Bit Status DEC.vi"("NomeStatus"=w1349) -> ("StatBit"=w1347:bool)
            n1031 = call "Bit Status AH.vi"("NomeStatus"=w1350) -> ("StatBit"=w1348:bool)
            n1032 = Or(x=w1348, y=w1347) -> (x .or. y?=w1346:bool)
            n1033 = case shown="True" w1346 {
              tunnel: [FALSE w1361] -> w1345
              tunnel: [w1351 w1362] -> w1336
              frame False {
                w1355 = u16 10 items=["Alarme", "Atencao", "Erro", "Ocupado", "Protecao", "Embreagem", "Tracking", "Var. Track", "Rápido", "Ligeiro", "Médio", "Lento", "Em movimento", ""] ("NomeStatus")
                w1354 = u16 10 items=["Alarme", "Atencao", "Erro", "Ocupado", "Protecao", "Embreagem", "Tracking", "Var. Track", "Rápido", "Ligeiro", "Médio", "Lento", "Em movimento", ""] ("NomeStatus")
                w1359 = u16 9 items=["Alarme", "Atencao", "Erro", "Ocupado", "Protecao", "Embreagem", "Tracking", "Var. Track", "Rápido", "Ligeiro", "Médio", "Lento", "Em movimento", ""] ("NomeStatus")
                w1360 = u16 9 items=["Alarme", "Atencao", "Erro", "Ocupado", "Protecao", "Embreagem", "Tracking", "Var. Track", "Rápido", "Ligeiro", "Médio", "Lento", "Em movimento", ""] ("NomeStatus")
                n1034 = call "Bit Status AH.vi"("NomeStatus"=w1360) -> ("StatBit"=w1358:bool)
                n1035 = call "Bit Status DEC.vi"("NomeStatus"=w1359) -> ("StatBit"=w1357:bool)
                n1036 = call "Bit Status AH.vi"("NomeStatus"=w1354) -> ("StatBit"=w1353:bool)
                n1037 = call "Bit Status DEC.vi"("NomeStatus"=w1355) -> ("StatBit"=w1352:bool)
                n1038 = Compound Arithmetic op=OR(w1358, w1357, w1353, w1352) -> (w1351:bool)
              }
              frame True {
                w1361 = TRUE
                n1039 = Not(x=w1361) -> (.not. x?=w1362:bool)
              }
            }
            "Mount Gross Movement" <- w1345
            "Mount Fine Movement" <- w1336
            n1040 = global read "Global_Telescopio.vi" "Bit RX Guider"() -> (w1344:bool)
            n1041 = global read "Global_Telescopio.vi" "Bit RX Aquis"() -> (w1343:bool)
            n1042 = case shown="True" w1344 {
              selector: w1344 -> [w1374 w1375]
              frame False {
                n1043 = local write "Auto guider Activity"(w1374) -> ()
              }
              frame True {
                # "Liga Led RX por 1 ciclo"
                n1044 = global write "Global_Telescopio.vi" "Bit RX Guider"(FALSE) -> ()
                "Auto guider Activity" <- w1375
              }
            }
            n1045 = case shown="True" w1343 {
              selector: w1343 -> [w1371 w1373]
              frame False {
                n1046 = local write "Data Acquisition Activity"(w1371) -> ()
              }
              frame True {
                # "Liga Led RX por 1 ciclo"
                n1047 = global write "Global_Telescopio.vi" "Bit RX Aquis"(FALSE) -> ()
                "Data Acquisition Activity" <- w1373
              }
            }
            n1048 = case shown="True" "News" {
              selector: "News" -> [_ w1367]
              frame False {
              }
              frame True {
                n1049 = flat-sequence {
                  tunnel: w1367 -> [w1368]
                  frame #0 {
                    n1050 = call "Monta_Mensagem.vi"("Zerar"=w1368) -> ()  [unwired: 2 in]
                  }
                  frame #1 {
                    n1051 = global write "Global_Telescopio.vi" "SYSTEM MESSAGES"("Novo controlador do foco do secundário, preciso e rápido.\nReformulação da comunicação do TCSPD, usando o protocolo ZeroMQ para publicar status. Arquivo LOG separado para erros de apontamento quando nome do objeto contrem \"@\". " ("SYSTEM MESSAGES")) -> ()
                  }
                }
              }
            }
            n1052 = global read "Global_Telescopio.vi" "SYSTEM MESSAGES"() -> (→"SYSTEM MESSAGES":string)
            n1053 = case shown="True" "Clear All Messages" {
              selector: "Clear All Messages" -> [_ w1370]
              frame False {
              }
              frame True {
                n1054 = call "Monta_Mensagem.vi"("Zerar"=w1370) -> ()  [unwired: 2 in]
              }
            }
            n1055 = local read "alarm Time"() -> (w1338:timestamp)
            n1056 = Get Date/Time In Seconds() -> (seconds since 1Jan1904=w1337:timestamp)
            n1057 = Greater?(x=w1337, y=w1338) -> (0:w1339:bool)
            n1058 = case shown="True" w1339 {
              frame False {
              }
              frame True {
                n1059 = local read "Flag Alarm"() -> (w1363:bool)
                n1060 = case shown="True" w1363 {
                  selector: w1363 -> [_ w1366]
                  frame False {
                  }
                  frame True {
                    n1061 = Not(x=w1366) -> (.not. x?=w1365:bool)
                    n1062 = property on="Mensage Alarme" class="Str"("Visible"=FALSE) -> ()  [unwired: 2 in, 2 out]
                    n1063 = local write "Flag Alarm"(w1365) -> ()
                  }
                }
              }
            }
          }
          frame #13 {
            w1381 = u16 3 items=["Alarme", "Atencao", "Erro", "Ocupado", "Protecao", "Embreagem", "Tracking", "Var. Track", "Rápido", "Ligeiro", "Médio", "Lento", "Em movimento", ""] ("NomeStatus")
            w1382 = u16 3 items=["Alarme", "Atencao", "Erro", "Ocupado", "Protecao", "Embreagem", "Tracking", "Var. Track", "Rápido", "Ligeiro", "Médio", "Lento", "Em movimento", ""] ("NomeStatus")
            # "PROCESSO AQUISIÇÃO"
            n1064 = global read "Global_Telescopio.vi" "Correção Aquis"() -> (w1377:bool)
            n1065 = call "Bit Status AH.vi"("NomeStatus"=w1382) -> ("StatBit"=w1379:bool)
            n1066 = call "Bit Status DEC.vi"("NomeStatus"=w1381) -> ("StatBit"=w1380:bool)
            n1067 = Not Or(1:w1380, 2:w1379) -> (0:w1378:bool)
            n1068 = Compound Arithmetic op=AND(w1377, w1378) -> (w1383:bool)
            n1069 = case shown="True" w1383 {
              frame False {
              }
              frame True {
                # "Reseta Flag do movimento de\n offset do Sist de Aquisição"
                n1070 = global read "Global_Telescopio.vi" "CorrecaoMin"() -> (w1389:dbl)
                n1071 = global read "Global_Telescopio.vi" "aquis_asc"() -> (w1388:dbl)
                n1072 = global read "Global_Telescopio.vi" "aquis_dec"() -> (w1391:dbl)
                n1073 = Absolute Value(x=w1391) -> (abs(x)=w1387:dbl)
                n1074 = global read "Global_Telescopio.vi" "CorrecaoMin"() -> (w1392:dbl)
                n1075 = global write "Global_Telescopio.vi" "Correção Aquis"(FALSE ("Correção Aquis")) -> ()
                n1076 = Absolute Value(x=w1388) -> (abs(x)=w1386:dbl)
                n1077 = Greater?(x=w1387, y=w1392) -> (0:w1393:bool)
                n1078 = Greater?(x=w1386, y=w1389) -> (0:w1390:bool)
                n1079 = case shown="True" w1390 {
                  tunnel: w1388 -> [_ w1394]
                  frame False {
                  }
                  frame True {
                    w1396 = u16 1 items=["ZERO", "AH", "DEC", "TUBO", "CUP"] ("Controlador")
                    # "PROCESSO MOVE TELESCÓPIO"
                    n1080 = call "Conversao Ms to Hora texto.vi"("TRUE=HORA\nFALSE=GRAU"=TRUE ("TRUE=HORA\nFALSE=GRAU"), "PrecDEC"=w1394) -> ("Hora/Graus Texto Decimal"=w1399:string)
                    n1081 = call "Monta Comando.vi"("Set Point"=w1399, "Comando"="MOVER_REL", "Dispositivo"="EIXO" ("Comando"), "Controlador"=w1396) -> ()  [unwired: 3 in, 3 out]
                  }
                }
                n1082 = case shown="True" w1393 {
                  tunnel: w1391 -> [_ w1400]
                  frame False {
                  }
                  frame True {
                    w1402 = u16 2 items=["ZERO", "AH", "DEC", "TUBO", "CUP"] ("Controlador")
                    # "PROCESSO MOVE TELESCÓPIO"
                    n1083 = call "Conversao Ms to Hora texto.vi"("TRUE=HORA\nFALSE=GRAU"=FALSE ("TRUE=HORA\nFALSE=GRAU"), "PrecDEC"=w1400) -> ("Hora/Graus Texto Decimal"=w1405:string)
                    n1084 = call "Monta Comando.vi"("Set Point"=w1405, "Comando"="MOVER_REL", "Dispositivo"="EIXO" ("Comando"), "Controlador"=w1402) -> ()  [unwired: 3 in, 3 out]
                  }
                }
                n1085 = global write "Global_Telescopio.vi" "AQ Offset Mov"(TRUE ("AQ Offset Mov")) -> ()
              }
            }
          }
          frame #14 {
            w1418 = "\r\n"
